vi "Logger-Log Info.vi"(11 "error in (no error)":errorcluster, 13 "Message":string) -> (15 "error out":errorcluster)   [LabVIEW 2020]
uses:
  Typedefs/Logger-Queue Data.ctl
  Typedefs/Logger-Action.ctl
  Typedefs/Logger-Level.ctl
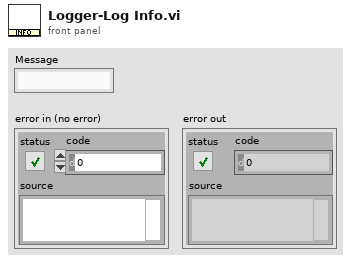
[diagram p1: front panel]
types:
  T1 = typedef "Logger-Level.ctl" = enum16{"Debug", "Info", "Warning", "Error", "Critical"}
  T2 = typedef "Logger-Action.ctl" = enum16{"None", "Init", "Add", "Quit"}
  T3 = typedef "Logger-Queue Data.ctl" = cluster{"Action":T2, "Level":T1, "Time":dbl, "Message":string}
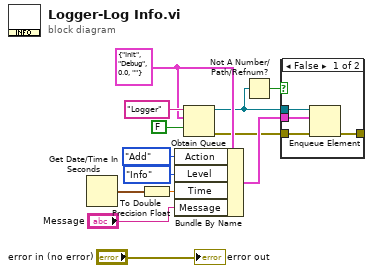
[diagram p0: block diagram]
diagram:
  w11 = T3 {"Action"=enum."Init", "Level"=enum."Debug", "Time"=0.0, "Message"=""} ("Trace Data")
  n1 = Get Date/Time In Seconds() -> (seconds since 1Jan1904=w7:timestamp)
  n2 = To Double Precision Float(number=w7) -> (double precision float=w8:dbl)
  n3 = Bundle By Name(cluster=w11, "Action"=Logger-Action."Add", "Level"=Logger-Level."Info", "Time"=w8, "Message"="Message") -> (w4:T3)
  n4 = Obtain Queue(name (unnamed)="Logger", element data type=w11, create if not found? (T)=FALSE) -> (queue out=w2:refnum<queue>, error out=w3:errorcluster)  [unwired: 2 in, 1 out]
  n5 = Not A Number/Path/Refnum?(number/path/refnum=w2) -> (NaN/Path/Refnum?=w1:bool)
  n6 = case shown="False" w1 {
    tunnel: w4 -> [w17 _]
    tunnel: w3 -> [w16 _]
    tunnel: w2 -> [w15 _]
    tunnel: [w14 _] -> _
    frame False {
      n7 = Enqueue Element(queue=w15, element=w17, error in (no error)=w16) -> (error out=w14:errorcluster)  [unwired: 1 in, 2 out]
    }
    frame True {
    }
  }
  "error out" <- "error in (no error)"
